vi "Stomach Model.vi"() -> ()   [LabVIEW 2018]
uses:
  <vilib>/Utility/file.llb/Read Delimited Spreadsheet (string).vi
  <vilib>/measure/mascope.llb/Cycle Average and RMS 1 chan.vi
  <vilib>/Analysis/NI_AAL_SigProc.lvlib
  <vilib>/measure/NI_MAPro.lvlib
panel:
  in  "?":bool
  in  "Select Next Ring":T1(ring)
  in  "Select Ring":T1(ring)
  out "Locations 8":dbl[](array[numeric])
  out "Locations 7":dbl[](array[numeric])
  out "Locations 6":dbl[](array[numeric])
  out "Locations 5":dbl[](array[numeric])
  out "Locations 4":dbl[](array[numeric])
  out "Locations 3":dbl[](array[numeric])
  out "Data":dbl[](array[numeric])
  out "Locations 2":dbl[](array[numeric])
  out "Locations":dbl[](array[numeric])
  out "Ring 7":i32[](array[numeric])
  out "Ring 6":i32[](array[numeric])
  out "Ring 5":i32[](array[numeric])
  out "Ring 4":i32[](array[numeric])
  out "Ring 3":i32[](array[numeric])
  out "Ring 2":i32[](array[numeric])
  out "Ring 1":i32[](array[numeric])
  out "Ring 0":i32[](array[numeric])
  out "Ring 7":i32[](graph)
  out "Ring 6":i32[](graph)
  out "Ring 5":i32[](graph)
  out "Ring 4":i32[](graph)
  out "Ring 3":i32[](graph)
  out "Ring 2":i32[](graph)
  out "Ring 1":i32[](graph)
  out "Ring 0":i32[](graph)
  in  "file path (dialog if empty)":path
  in  "stop":bool
  out "Ring 4 Start":u32
  out "Ring 7 Start":u32
  out "Ring 6 Start":u32
  out "Ring 5 Start":u32
  out "Ring 3 Start":u32
  out "Ring 2 Start":u32
  out "Ring 1 Start":u32
  out "Ring 0 Start":u32
  out "Run Time":u32
  in  "Time Delay 2":u32
  in  "Time Delay 1":u32
  in  "Time Delay 0":u32
  out "Ring 7":bool
  out "Ring 6":bool
  out "Ring 5":bool
  out "Ring 4":bool
  out "Ring 3":bool
  out "Ring 2":bool
  out "Ring 1":bool
  out "Time":u32
  out "Ring 0":bool
  # "Pacemaker"
  # "Stomach Model"
  # "Ring 0"
  # "Ring 1"
  # "Ring 2"
  # "Corpus"
  # "Ring 3"
  # "Ring 4"
  # "Ring 5"
  # "Antrum"
  # "Ring 6"
  # "Ring 7"
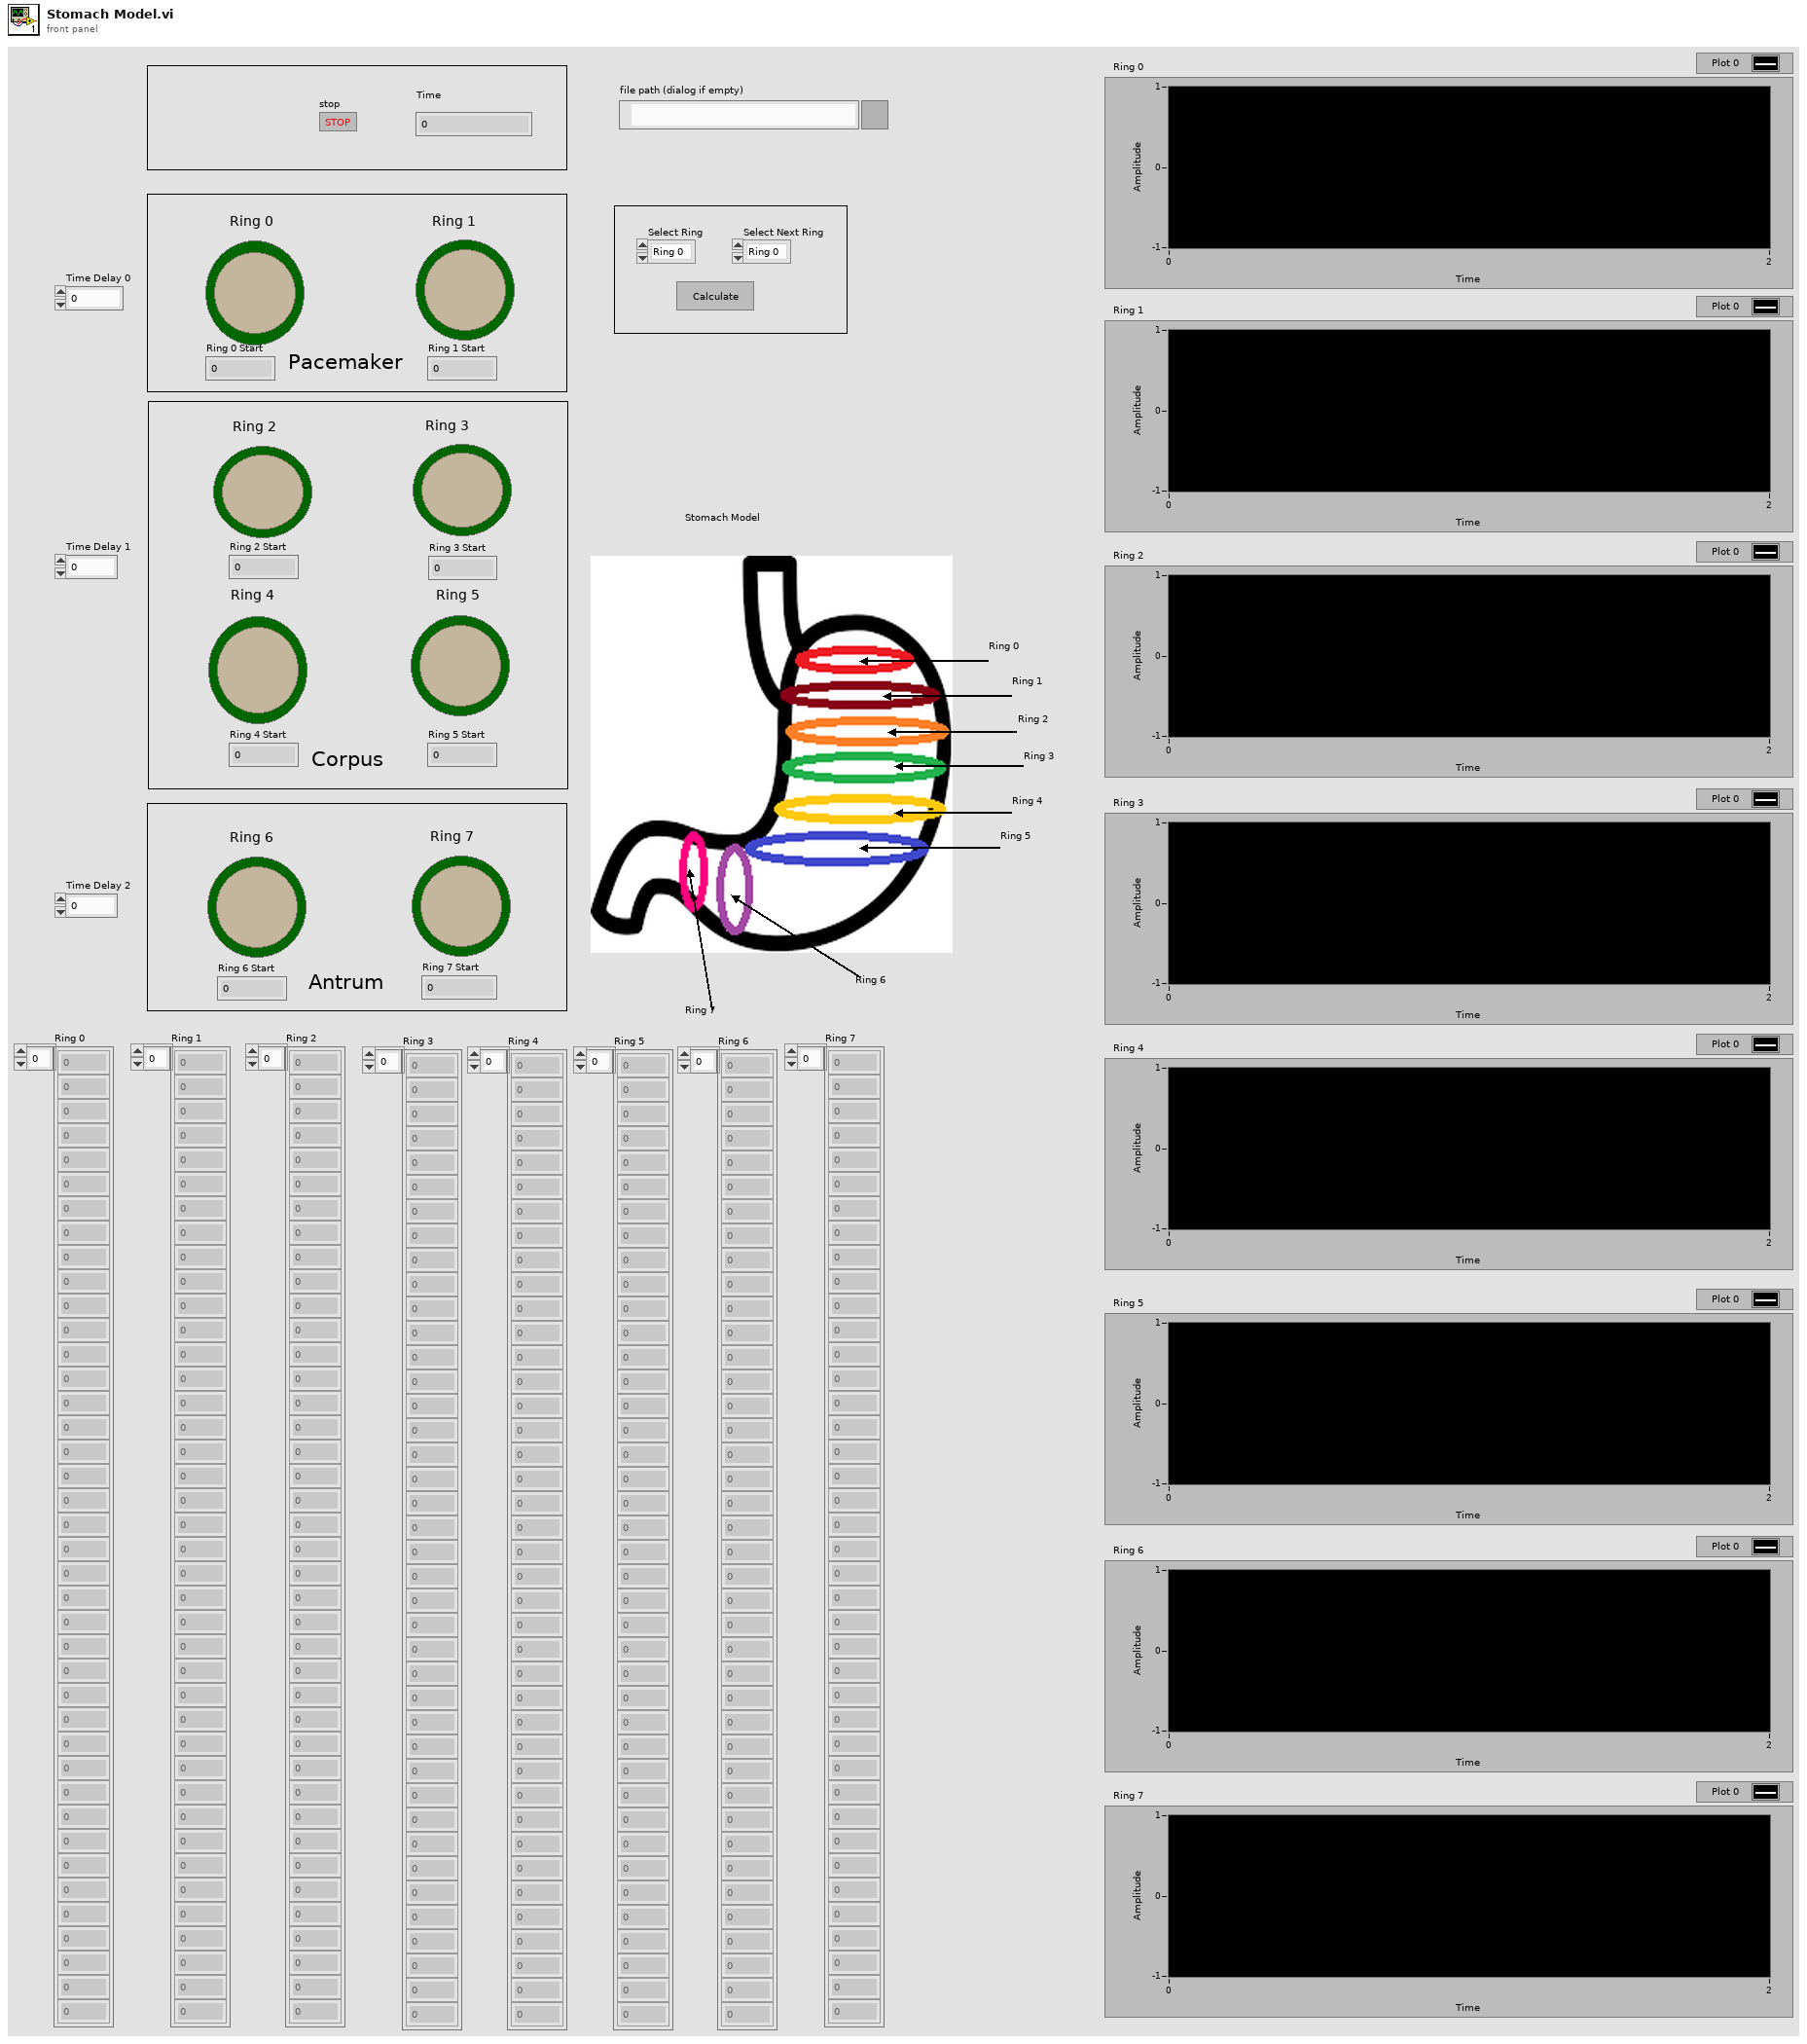
[diagram p1: front panel]
types:
  T1 = enum16{"Ring 0", "Ring 1", "Ring 2", "Ring 3", "Ring 4", "Ring 5", "Ring 6", "Ring 7"}
  T2 = cluster{"high ref level":dbl, "mid ref level":dbl, "low ref level":dbl, "ref units":u16}
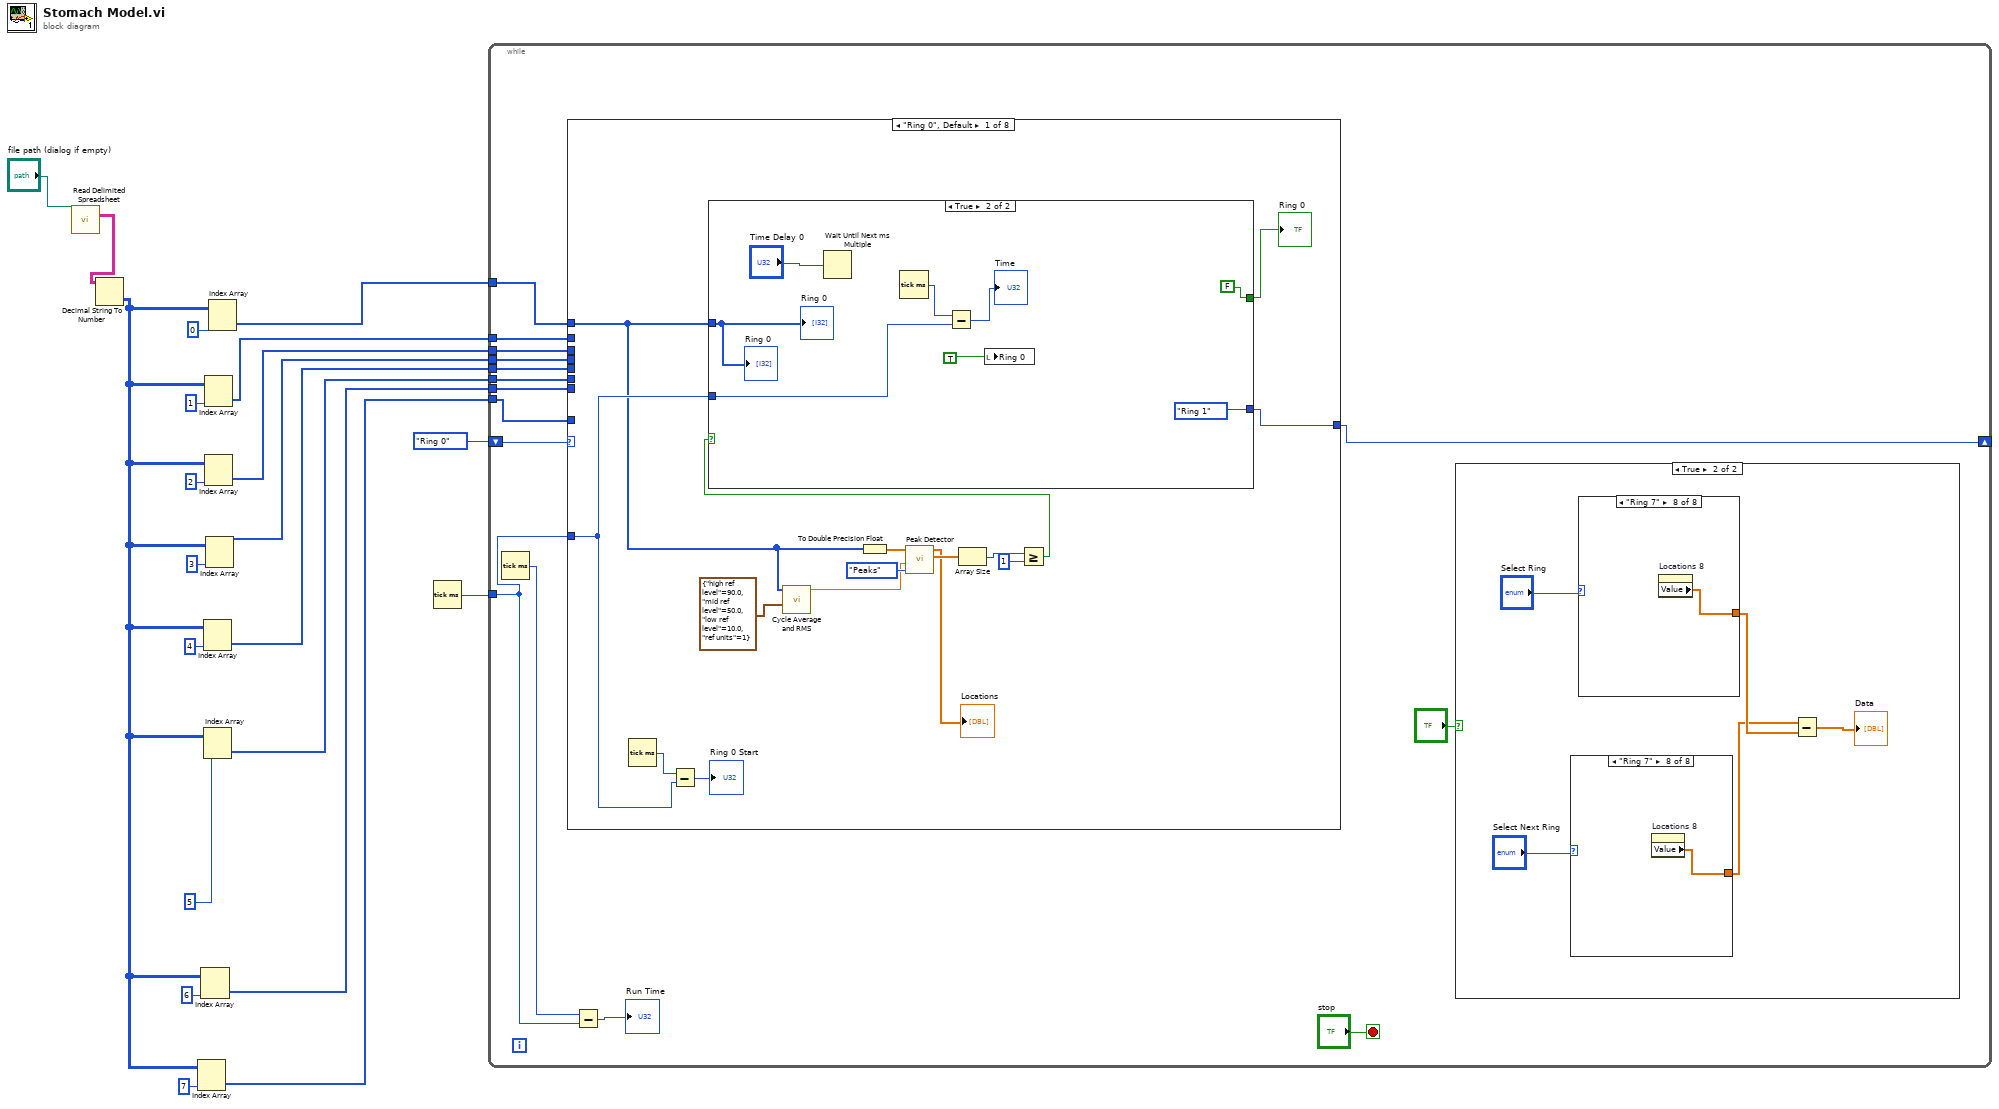
[diagram p0: block diagram]
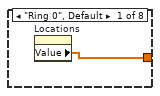
[diagram p3: hidden frame]
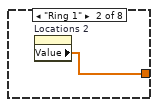
[diagram p4: hidden frame]
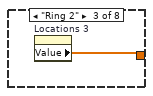
[diagram p5: hidden frame]
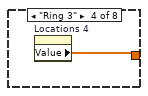
[diagram p6: hidden frame]
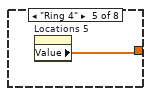
[diagram p7: hidden frame]
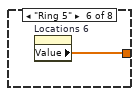
[diagram p8: hidden frame]
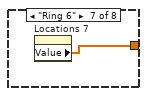
[diagram p9: hidden frame]
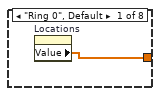
[diagram p10: hidden frame]
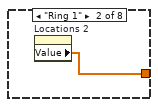
[diagram p11: hidden frame]
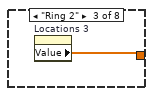
[diagram p12: hidden frame]
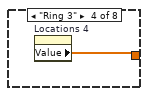
[diagram p13: hidden frame]
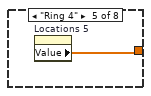
[diagram p14: hidden frame]
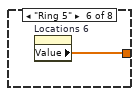
[diagram p15: hidden frame]
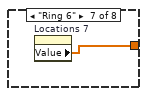
[diagram p16: hidden frame]
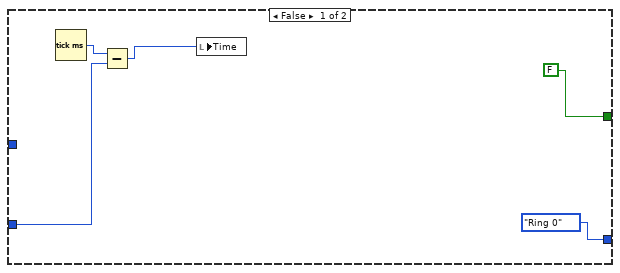
[diagram p17: hidden frame]
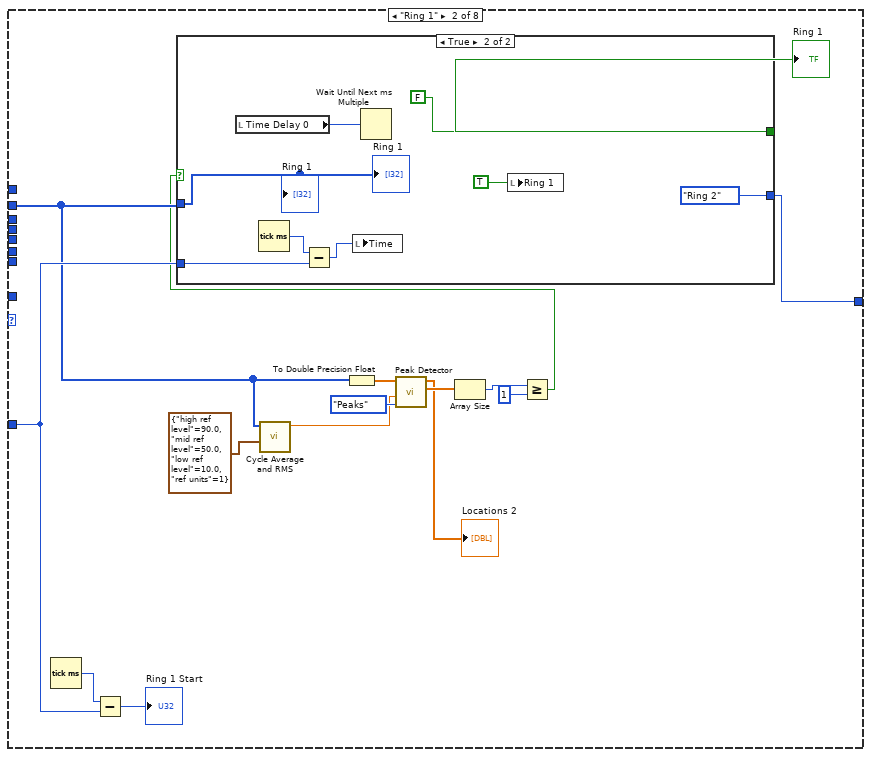
[diagram p18: hidden frame]
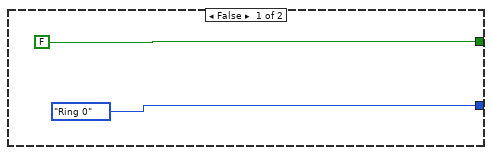
[diagram p19: hidden frame]
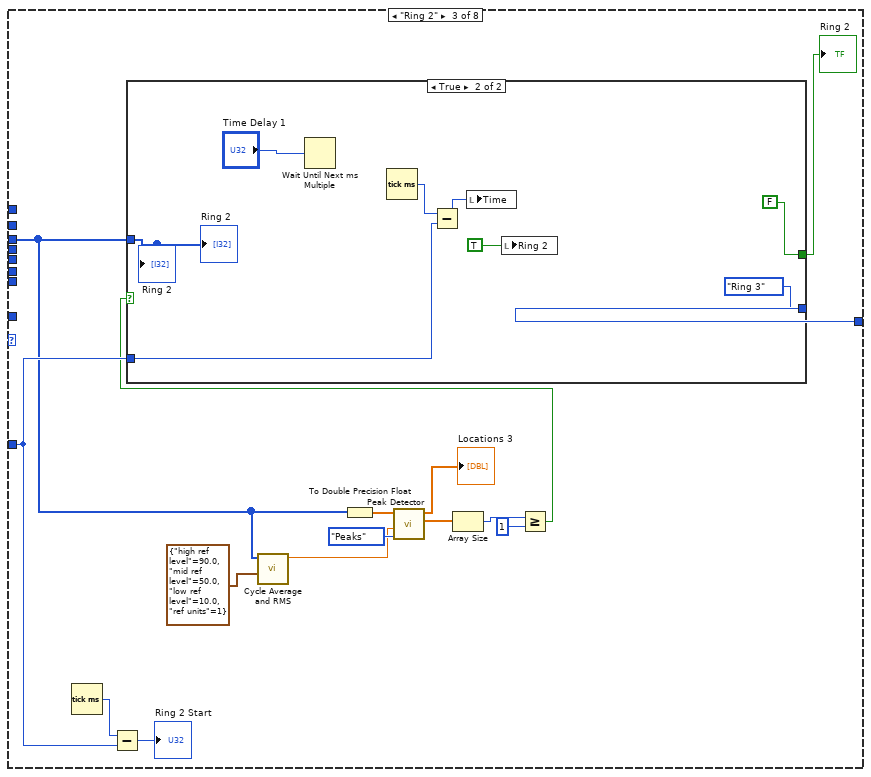
[diagram p20: hidden frame]
diagram:
  n1 = call-poly <vilib>:"Read Delimited Spreadsheet.vi"("file path (dialog if empty)"="file path (dialog if empty)") -> ("all rows"=w17:string[][])  [unwired: 9 in, 5 out]
  n2 = Decimal String To Number(string=w17) -> (number=w12:i32[][])  [unwired: 2 in, 1 out]
  n3 = Index Array(array=w12, index (col)=7 ("disabled index (col)")) -> (element=w1:i32[])  [unwired: 1 in]
  n4 = Index Array(array=w12, index (col)=6 ("disabled index (col)")) -> (element=w2:i32[])  [unwired: 1 in]
  n5 = Index Array(array=w12, index (col)=4 ("disabled index (col)")) -> (element=w4:i32[])  [unwired: 1 in]
  n6 = Index Array(array=w12, index (col)=5 ("disabled index (col)")) -> (element=w3:i32[])  [unwired: 1 in]
  n7 = Index Array(array=w12, index (col)=1 ("disabled index (col)")) -> (element=w7:i32[])  [unwired: 1 in]
  n8 = Index Array(array=w12, index (col)=2 ("disabled index (col)")) -> (element=w6:i32[])  [unwired: 1 in]
  n9 = Index Array(array=w12, index (col)=3 ("disabled index (col)")) -> (element=w5:i32[])  [unwired: 1 in]
  n10 = Index Array(array=w12, index (col)=0 ("disabled index (col)")) -> (element=w8:i32[])  [unwired: 1 in]
  n11 = Tick Count (ms)() -> (millisecond timer value=w20:u32)
  n12 = while {
    shift-right: [w35] -> _
    shift-left: T1."Ring 0" ("Enum") -> [w36]
    tunnel: w20 -> [w32]
    tunnel: w8 -> [w30]
    tunnel: w7 -> [w29]
    tunnel: w6 -> [w28]
    tunnel: w5 -> [w27]
    tunnel: w4 -> [w26]
    tunnel: w3 -> [w25]
    tunnel: w2 -> [w24]
    tunnel: w1 -> [w23]
    stop <- "stop" stop-if-true
    n13 = Tick Count (ms)() -> (millisecond timer value=w34:u32)
    n14 = case shown="\"Ring 0\", Default" w36 {
      tunnel: [w71 w99 w124 w149 w174 w199 w224 w249] -> w35
      tunnel: w32 -> [w69 w97 w121 w146 w171 w196 w221 w246]
      tunnel: w30 -> [w60 _ _ _ _ _ _ _]
      tunnel: w29 -> [_ w88 _ _ _ _ _ _]
      tunnel: w28 -> [_ _ w113 _ _ _ _ _]
      tunnel: w27 -> [_ _ _ w138 _ _ _ _]
      tunnel: w26 -> [_ _ _ _ w163 _ _ _]
      tunnel: w25 -> [_ _ _ _ _ w188 _ _]
      tunnel: w24 -> [_ _ _ _ _ _ w213 _]
      tunnel: w23 -> [_ _ _ _ _ _ _ w238]
      frame "Ring 0", Default {
        n15 = Tick Count (ms)() -> (millisecond timer value=w70:u32)
        n16 = Subtract(x=w70, y=w69) -> (x-y=→"Ring 0 Start":u32)
        n17 = call-poly <vilib>:"Cycle Average and RMS.vi"("reference levels"=T2 {"high ref level"=90.0, "mid ref level"=50.0, "low ref level"=10.0, "ref units"=1}, "signal in"=w60) -> ("cycle average"=w61:dbl)  [unwired: 6 in, 3 out]
        n18 = To Double Precision Float(number=w60) -> (double precision float=w67:dbl[])
        n19 = call <vilib>:"Peak Detector.vi"("peaks/valleys"=enum32{"Peaks", "Valleys"}."Peaks", "width"=w61, "X"=w67) -> ("Amplitudes"=w66:dbl[], "Locations"=→"Locations":dbl[])  [unwired: 4 in, 3 out]
        n20 = Array Size(array=w66) -> (size(s)=w65:i32)
        n21 = Greater Or Equal?(x=w65, y=1) -> (x >= y?=w59:bool)
        n22 = case shown="True" w59 {
          tunnel: [FALSE FALSE] -> w72
          tunnel: [T1."Ring 0" ("Enum") T1."Ring 1" ("Enum")] -> w71
          tunnel: w69 -> [w74 w80]
          tunnel: w60 -> [_ w78]
          frame False {
            n23 = Tick Count (ms)() -> (millisecond timer value=w75:u32)
            n24 = Subtract(x=w75, y=w74) -> (x-y=w73:u32)
            n25 = local write "Time"(w73) -> ()
          }
          frame True {
            n26 = Wait Until Next ms Multiple(millisecond multiple="Time Delay 0") -> ()  [unwired: 1 out]
            n27 = Tick Count (ms)() -> (millisecond timer value=w81:u32)
            n28 = Subtract(x=w81, y=w80) -> (x-y=→"Time":u32)
            n29 = local write "Ring 0"(TRUE) -> ()
            "Ring 0" <- w78
            "Ring 0" <- w78
          }
        }
        "Ring 0" <- w72
      }
      frame "Ring 1" {
        n30 = Tick Count (ms)() -> (millisecond timer value=w96:u32)
        n31 = Subtract(x=w96, y=w97) -> (x-y=→"Ring 1 Start":u32)
        n32 = call-poly <vilib>:"Cycle Average and RMS.vi"("reference levels"=T2 {"high ref level"=90.0, "mid ref level"=50.0, "low ref level"=10.0, "ref units"=1}, "signal in"=w88) -> ("cycle average"=w89:dbl)  [unwired: 6 in, 3 out]
        n33 = To Double Precision Float(number=w88) -> (double precision float=w95:dbl[])
        n34 = call <vilib>:"Peak Detector.vi"("peaks/valleys"=enum32{"Peaks", "Valleys"}."Peaks", "width"=w89, "X"=w95) -> ("Amplitudes"=w94:dbl[], "Locations"=→"Locations 2":dbl[])  [unwired: 4 in, 3 out]
        n35 = Array Size(array=w94) -> (size(s)=w93:i32)
        n36 = Greater Or Equal?(x=w93, y=1) -> (x >= y?=w87:bool)
        n37 = case shown="True" w87 {
          tunnel: [T1."Ring 0" ("Enum") T1."Ring 2" ("Enum")] -> w99
          tunnel: [FALSE FALSE] -> w100
          tunnel: w97 -> [_ w105]
          tunnel: w88 -> [_ w103]
          frame False {
          }
          frame True {
            n38 = local read "Time Delay 0"() -> (w107:u32)
            n39 = Tick Count (ms)() -> (millisecond timer value=w106:u32)
            n40 = Subtract(x=w106, y=w105) -> (x-y=w104:u32)
            n41 = local write "Time"(w104) -> ()
            n42 = Wait Until Next ms Multiple(millisecond multiple=w107) -> ()  [unwired: 1 out]
            n43 = local write "Ring 1"(TRUE ("Boolean 2")) -> ()
            "Ring 1" <- w103
            "Ring 1" <- w103
          }
        }
        "Ring 1" <- w100
      }
      frame "Ring 2" {
        n44 = Tick Count (ms)() -> (millisecond timer value=w123:u32)
        n45 = Subtract(x=w123, y=w121) -> (x-y=→"Ring 2 Start":u32)
        n46 = call-poly <vilib>:"Cycle Average and RMS.vi"("reference levels"=T2 {"high ref level"=90.0, "mid ref level"=50.0, "low ref level"=10.0, "ref units"=1}, "signal in"=w113) -> ("cycle average"=w114:dbl)  [unwired: 6 in, 3 out]
        n47 = To Double Precision Float(number=w113) -> (double precision float=w120:dbl[])
        n48 = call <vilib>:"Peak Detector.vi"("peaks/valleys"=enum32{"Peaks", "Valleys"}."Peaks", "width"=w114, "X"=w120) -> ("Amplitudes"=w119:dbl[], "Locations"=→"Locations 3":dbl[])  [unwired: 4 in, 3 out]
        n49 = Array Size(array=w119) -> (size(s)=w118:i32)
        n50 = Greater Or Equal?(x=w118, y=1) -> (x >= y?=w112:bool)
        n51 = case shown="True" w112 {
          tunnel: [FALSE FALSE] -> w125
          tunnel: [T1."Ring 0" ("Enum") T1."Ring 3" ("Enum")] -> w124
          tunnel: w121 -> [_ w129]
          tunnel: w113 -> [_ w128]
          frame False {
          }
          frame True {
            n52 = Wait Until Next ms Multiple(millisecond multiple="Time Delay 1") -> ()  [unwired: 1 out]
            n53 = Tick Count (ms)() -> (millisecond timer value=w130:u32)
            n54 = Subtract(x=w130, y=w129) -> (x-y=w131:u32)
            n55 = local write "Time"(w131) -> ()
            n56 = local write "Ring 2"(TRUE ("Boolean 2")) -> ()
            "Ring 2" <- w128
            "Ring 2" <- w128
          }
        }
        "Ring 2" <- w125
      }
      frame "Ring 3" {
        n57 = Tick Count (ms)() -> (millisecond timer value=w148:u32)
        n58 = Subtract(x=w148, y=w146) -> (x-y=→"Ring 3 Start":u32)
        n59 = call-poly <vilib>:"Cycle Average and RMS.vi"("reference levels"=T2 {"high ref level"=90.0, "mid ref level"=50.0, "low ref level"=10.0, "ref units"=1}, "signal in"=w138) -> ("cycle average"=w139:dbl)  [unwired: 6 in, 3 out]
        n60 = To Double Precision Float(number=w138) -> (double precision float=w145:dbl[])
        n61 = call <vilib>:"Peak Detector.vi"("peaks/valleys"=enum32{"Peaks", "Valleys"}."Peaks", "width"=w139, "X"=w145) -> ("Amplitudes"=w144:dbl[], "Locations"=→"Locations 4":dbl[])  [unwired: 4 in, 3 out]
        n62 = Array Size(array=w144) -> (size(s)=w143:i32)
        n63 = Greater Or Equal?(x=w143, y=1) -> (x >= y?=w137:bool)
        n64 = case shown="True" w137 {
          tunnel: [FALSE FALSE] -> w150
          tunnel: [T1."Ring 0" ("Enum") T1."Ring 4" ("Enum")] -> w149
          tunnel: w146 -> [_ w154]
          tunnel: w138 -> [_ w153]
          frame False {
          }
          frame True {
            n65 = Tick Count (ms)() -> (millisecond timer value=w156:u32)
            n66 = local read "Time Delay 1"() -> (w157:u32)
            n67 = Subtract(x=w156, y=w154) -> (x-y=w155:u32)
            n68 = local write "Time"(w155) -> ()
            n69 = Wait Until Next ms Multiple(millisecond multiple=w157) -> ()  [unwired: 1 out]
            n70 = local write "Ring 3"(TRUE ("Boolean 2")) -> ()
            "Ring 3" <- w153
            "Ring 3" <- w153
          }
        }
        "Ring 3" <- w150
      }
      frame "Ring 4" {
        n71 = Tick Count (ms)() -> (millisecond timer value=w173:u32)
        n72 = Subtract(x=w173, y=w171) -> (x-y=→"Ring 4 Start":u32)
        n73 = call-poly <vilib>:"Cycle Average and RMS.vi"("reference levels"=T2 {"high ref level"=90.0, "mid ref level"=50.0, "low ref level"=10.0, "ref units"=1}, "signal in"=w163) -> ("cycle average"=w164:dbl)  [unwired: 6 in, 3 out]
        n74 = To Double Precision Float(number=w163) -> (double precision float=w170:dbl[])
        n75 = call <vilib>:"Peak Detector.vi"("peaks/valleys"=enum32{"Peaks", "Valleys"}."Peaks", "width"=w164, "X"=w170) -> ("Amplitudes"=w169:dbl[], "Locations"=→"Locations 5":dbl[])  [unwired: 4 in, 3 out]
        n76 = Array Size(array=w169) -> (size(s)=w168:i32)
        n77 = Greater Or Equal?(x=w168, y=1) -> (x >= y?=w162:bool)
        n78 = case shown="True" w162 {
          tunnel: [FALSE FALSE] -> w175
          tunnel: [T1."Ring 0" ("Enum") T1."Ring 5" ("Enum")] -> w174
          tunnel: w171 -> [_ w180]
          tunnel: w163 -> [_ w178]
          frame False {
          }
          frame True {
            n79 = local read "Time Delay 1"() -> (w182:u32)
            n80 = Wait Until Next ms Multiple(millisecond multiple=w182) -> ()  [unwired: 1 out]
            n81 = Tick Count (ms)() -> (millisecond timer value=w181:u32)
            n82 = Subtract(x=w181, y=w180) -> (x-y=w179:u32)
            n83 = local write "Time"(w179) -> ()
            n84 = local write "Ring 4"(TRUE ("Boolean 2")) -> ()
            "Ring 4" <- w178
            "Ring 4" <- w178
          }
        }
        "Ring 4" <- w175
      }
      frame "Ring 5" {
        n85 = Tick Count (ms)() -> (millisecond timer value=w198:u32)
        n86 = Subtract(x=w198, y=w196) -> (x-y=→"Ring 5 Start":u32)
        n87 = call-poly <vilib>:"Cycle Average and RMS.vi"("reference levels"=T2 {"high ref level"=90.0, "mid ref level"=50.0, "low ref level"=10.0, "ref units"=1}, "signal in"=w188) -> ("cycle average"=w189:dbl)  [unwired: 6 in, 3 out]
        n88 = To Double Precision Float(number=w188) -> (double precision float=w195:dbl[])
        n89 = call <vilib>:"Peak Detector.vi"("peaks/valleys"=enum32{"Peaks", "Valleys"}."Peaks", "width"=w189, "X"=w195) -> ("Amplitudes"=w194:dbl[], "Locations"=→"Locations 6":dbl[])  [unwired: 4 in, 3 out]
        n90 = Array Size(array=w194) -> (size(s)=w193:i32)
        n91 = Greater Or Equal?(x=w193, y=1) -> (x >= y?=w187:bool)
        n92 = case shown="True" w187 {
          tunnel: [T1."Ring 0" ("Enum") T1."Ring 6" ("Enum")] -> w199
          tunnel: [FALSE FALSE] -> w200
          tunnel: w196 -> [_ w205]
          tunnel: w188 -> [_ w203]
          frame False {
          }
          frame True {
            n93 = local read "Time Delay 1"() -> (w207:u32)
            n94 = Wait Until Next ms Multiple(millisecond multiple=w207) -> ()  [unwired: 1 out]
            n95 = Tick Count (ms)() -> (millisecond timer value=w206:u32)
            n96 = Subtract(x=w206, y=w205) -> (x-y=w204:u32)
            n97 = local write "Time"(w204) -> ()
            n98 = local write "Ring 5"(TRUE ("Boolean 2")) -> ()
            "Ring 5" <- w203
            "Ring 5" <- w203
          }
        }
        "Ring 5" <- w200
      }
      frame "Ring 6" {
        n99 = Tick Count (ms)() -> (millisecond timer value=w223:u32)
        n100 = Subtract(x=w223, y=w221) -> (x-y=→"Ring 6 Start":u32)
        n101 = call-poly <vilib>:"Cycle Average and RMS.vi"("reference levels"=T2 {"high ref level"=90.0, "mid ref level"=50.0, "low ref level"=10.0, "ref units"=1}, "signal in"=w213) -> ("cycle average"=w214:dbl)  [unwired: 6 in, 3 out]
        n102 = To Double Precision Float(number=w213) -> (double precision float=w220:dbl[])
        n103 = call <vilib>:"Peak Detector.vi"("peaks/valleys"=enum32{"Peaks", "Valleys"}."Peaks", "width"=w214, "X"=w220) -> ("Amplitudes"=w219:dbl[], "Locations"=→"Locations 7":dbl[])  [unwired: 4 in, 3 out]
        n104 = Array Size(array=w219) -> (size(s)=w218:i32)
        n105 = Greater Or Equal?(x=w218, y=1) -> (x >= y?=w212:bool)
        n106 = case shown="True" w212 {
          tunnel: [T1."Ring 0" ("Enum") T1."Ring 7" ("Enum")] -> w224
          tunnel: [FALSE FALSE] -> w225
          tunnel: w221 -> [_ w230]
          tunnel: w213 -> [_ w228]
          frame False {
          }
          frame True {
            n107 = Tick Count (ms)() -> (millisecond timer value=w231:u32)
            n108 = Wait Until Next ms Multiple(millisecond multiple="Time Delay 2") -> ()  [unwired: 1 out]
            n109 = Subtract(x=w231, y=w230) -> (x-y=w229:u32)
            n110 = local write "Time"(w229) -> ()
            n111 = local write "Ring 6"(TRUE ("Boolean 2")) -> ()
            "Ring 6" <- w228
            "Ring 6" <- w228
          }
        }
        "Ring 6" <- w225
      }
      frame "Ring 7" {
        n112 = Tick Count (ms)() -> (millisecond timer value=w248:u32)
        n113 = Subtract(x=w248, y=w246) -> (x-y=→"Ring 7 Start":u32)
        n114 = call-poly <vilib>:"Cycle Average and RMS.vi"("reference levels"=T2 {"high ref level"=90.0, "mid ref level"=50.0, "low ref level"=10.0, "ref units"=1}, "signal in"=w238) -> ("cycle average"=w239:dbl)  [unwired: 6 in, 3 out]
        n115 = To Double Precision Float(number=w238) -> (double precision float=w245:dbl[])
        n116 = call <vilib>:"Peak Detector.vi"("peaks/valleys"=enum32{"Peaks", "Valleys"}."Peaks", "width"=w239, "X"=w245) -> ("Amplitudes"=w244:dbl[], "Locations"=→"Locations 8":dbl[])  [unwired: 4 in, 3 out]
        n117 = Array Size(array=w244) -> (size(s)=w243:i32)
        n118 = Greater Or Equal?(x=w243, y=1) -> (x >= y?=w237:bool)
        n119 = case shown="True" w237 {
          tunnel: [FALSE FALSE] -> w250
          tunnel: [T1."Ring 0" ("Enum") T1."Ring 0" ("Enum")] -> w249
          tunnel: w246 -> [_ w256]
          tunnel: w238 -> [_ w253]
          frame False {
          }
          frame True {
            n120 = local read "Time Delay 2"() -> (w257:u32)
            n121 = Wait Until Next ms Multiple(millisecond multiple=w257) -> ()  [unwired: 1 out]
            n122 = Tick Count (ms)() -> (millisecond timer value=w255:u32)
            n123 = Subtract(x=w255, y=w256) -> (x-y=w254:u32)
            n124 = local write "Time"(w254) -> ()
            n125 = local write "Ring 7"(TRUE ("Boolean 2")) -> ()
            "Ring 7" <- w253
            "Ring 7" <- w253
          }
        }
        "Ring 7" <- w250
      }
    }
    n126 = Subtract(x=w34, y=w32) -> (x-y=→"Run Time":u32)
    n127 = case shown="True" "?" {
      frame False {
      }
      frame True {
        n128 = case shown="\"Ring 7\"" "Select Next Ring" {
          tunnel: [w42 w43 w44 w45 w46 w47 w48 w49] -> w37
          frame "Ring 0", Default {
            n129 = property on="Locations" class="Arr (strict)"() -> ("Value"=w42:dbl[])  [unwired: 2 in, 2 out]
          }
          frame "Ring 1" {
            n130 = property on="Locations 2" class="Arr (strict)"() -> ("Value"=w43:dbl[])  [unwired: 2 in, 2 out]
          }
          frame "Ring 2" {
            n131 = property on="Locations 3" class="Arr (strict)"() -> ("Value"=w44:dbl[])  [unwired: 2 in, 2 out]
          }
          frame "Ring 3" {
            n132 = property on="Locations 4" class="Arr (strict)"() -> ("Value"=w45:dbl[])  [unwired: 2 in, 2 out]
          }
          frame "Ring 4" {
            n133 = property on="Locations 5" class="Arr (strict)"() -> ("Value"=w46:dbl[])  [unwired: 2 in, 2 out]
          }
          frame "Ring 5" {
            n134 = property on="Locations 6" class="Arr (strict)"() -> ("Value"=w47:dbl[])  [unwired: 2 in, 2 out]
          }
          frame "Ring 6" {
            n135 = property on="Locations 7" class="Arr (strict)"() -> ("Value"=w48:dbl[])  [unwired: 2 in, 2 out]
          }
          frame "Ring 7" {
            n136 = property on="Locations 8" class="Arr (strict)"() -> ("Value"=w49:dbl[])  [unwired: 2 in, 2 out]
          }
        }
        n137 = case shown="\"Ring 7\"" "Select Ring" {
          tunnel: [w50 w51 w52 w53 w54 w55 w56 w57] -> w38
          frame "Ring 0", Default {
            n138 = property on="Locations" class="Arr (strict)"() -> ("Value"=w50:dbl[])  [unwired: 2 in, 2 out]
          }
          frame "Ring 1" {
            n139 = property on="Locations 2" class="Arr (strict)"() -> ("Value"=w51:dbl[])  [unwired: 2 in, 2 out]
          }
          frame "Ring 2" {
            n140 = property on="Locations 3" class="Arr (strict)"() -> ("Value"=w52:dbl[])  [unwired: 2 in, 2 out]
          }
          frame "Ring 3" {
            n141 = property on="Locations 4" class="Arr (strict)"() -> ("Value"=w53:dbl[])  [unwired: 2 in, 2 out]
          }
          frame "Ring 4" {
            n142 = property on="Locations 5" class="Arr (strict)"() -> ("Value"=w54:dbl[])  [unwired: 2 in, 2 out]
          }
          frame "Ring 5" {
            n143 = property on="Locations 6" class="Arr (strict)"() -> ("Value"=w55:dbl[])  [unwired: 2 in, 2 out]
          }
          frame "Ring 6" {
            n144 = property on="Locations 7" class="Arr (strict)"() -> ("Value"=w56:dbl[])  [unwired: 2 in, 2 out]
          }
          frame "Ring 7" {
            n145 = property on="Locations 8" class="Arr (strict)"() -> ("Value"=w57:dbl[])  [unwired: 2 in, 2 out]
          }
        }
        n146 = Subtract(x=w37, y=w38) -> (x-y=→"Data":dbl[])
      }
    }
  }
